vi "Convert Variants To Contents.vi"(8 "error in":errorcluster, 11 "ExcuseNote":variant[](array[variant])) -> (0 "error out":errorcluster, 3 "ExcuseNote(\"\")":string[](array[string]))   [LabVIEW 2015, in "ExcuseNotesHandler.lvclass"]
uses:
  ExcuseNotesHandler.lvclass
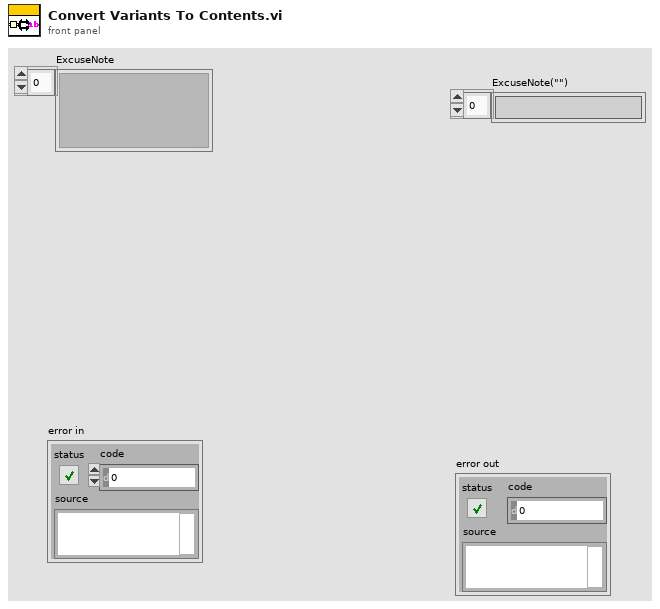
[diagram p1: front panel]
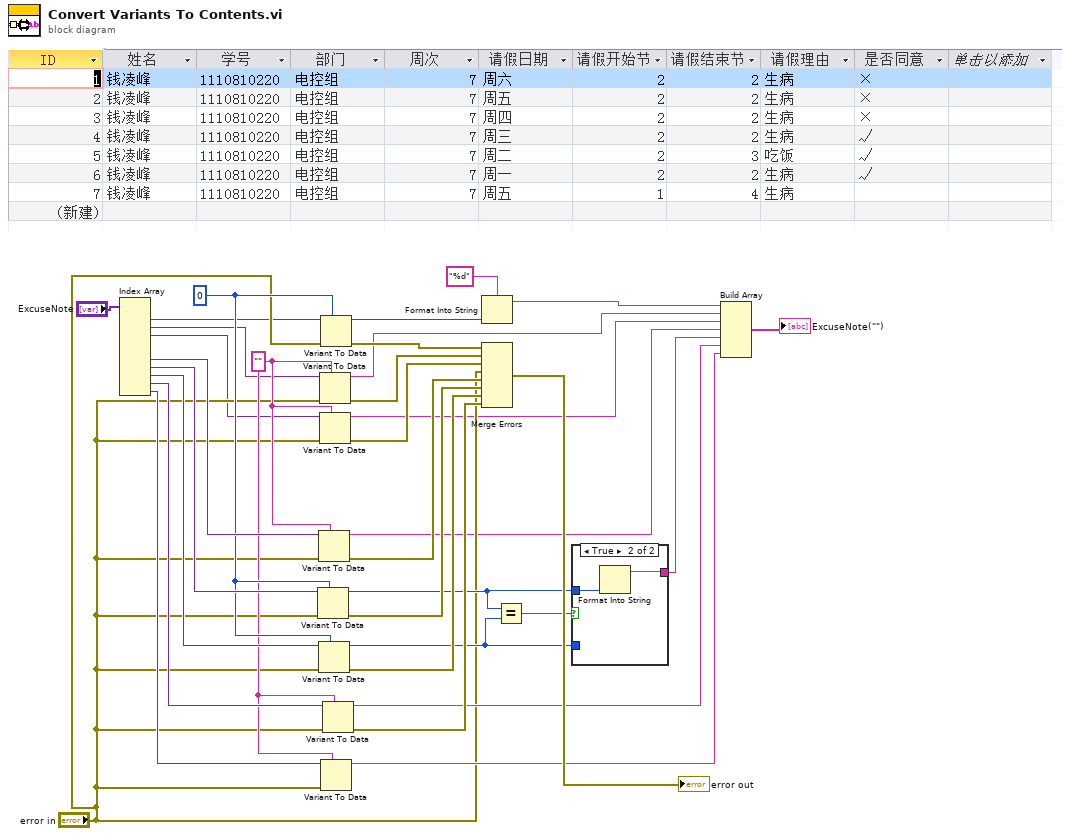
[diagram p0: block diagram]
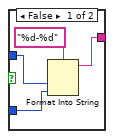
[diagram p2: hidden frame]
diagram:
  w7 = ""
  w29 = 0
  n1 = Index Array(array="ExcuseNote") -> (element #1=w3:variant, element #2=w2:variant, element #3=w1:variant, element #6=w32:variant, element #7=w31:variant, element #8=w30:variant, element #9=w28:variant, element #10=w9:variant)  [unwired: 10 in, 2 out]
  n2 = Variant To Data(error in="error in", type=w29, Variant=w31) -> (data=w14:i32, error out=w23:errorcluster)
  n3 = Variant To Data(error in="error in", type=w7, Variant=w32) -> (data=w5:string, error out=w24:errorcluster)
  n4 = Variant To Data(error in="error in", type=w29, Variant=w30) -> (data=w13:i32, error out=w22:errorcluster)
  n5 = Variant To Data(error in="error in", type=w7, Variant=w2) -> (data=w15:string, error out=w26:errorcluster)
  n6 = Variant To Data(error in="error in", type=w7, Variant=w1) -> (data=w4:string, error out=w25:errorcluster)
  n7 = Variant To Data(error in="error in", type=w29, Variant=w3) -> (data=w18:i32, error out=w27:errorcluster)
  n8 = Variant To Data(error in="error in", type=w7, Variant=w9) -> (data=w8:string)  [unwired: 1 out]
  n9 = Variant To Data(error in="error in", type=w7, Variant=w28) -> (data=w11:string, error out=w21:errorcluster)
  n10 = Format Into String(format string="%d", w18) -> (resulting string=w16:string)  [unwired: 2 in, 1 out]
  n11 = Merge Errors(w27, w26, w25, "error in", w24, w23, w22, w21) -> (→"error out":errorcluster)
  n12 = Equal?(x=w14, y=w13) -> (x = y?=w19:bool)
  n13 = case shown="True" w19 {
    tunnel: w14 -> [w36 w39]
    tunnel: w13 -> [w35 _]
    tunnel: [w34 w38] -> w12
    frame False {
      n14 = Format Into String(format string="%d-%d", w36, w35) -> (resulting string=w34:string)  [unwired: 2 in, 1 out]
    }
    frame True {
      n15 = Format Into String(w39) -> (resulting string=w38:string)  [unwired: 3 in, 1 out]
    }
  }
  n16 = Build Array(w16, w15, w4, w5, w12, w11, w8) -> (→"ExcuseNote(\"\")":string[])
